vi "Adjust SMU Meas Sense.vi"(7 "Pins":string[](array[string]), 8 "error in (no error)":errorcluster, 10 "Set_Meas_Sense":i32(ring)=1008 items=["Local"=1008, "Remote"=1009], 11 "Semiconductor Module Context":T1) -> (0 "error out":errorcluster, 1 "Measurement:Sense":i32(ring)=1008 items=["Local"=1008, "Remote"=1009], 3 "Semiconductor Module Context Out":T1)   [LabVIEW 2013]
uses:
  <vilib>/NI_TestStand_SemiconductorModule/NI_TestStand_Semiconductor_Module.lvlibp/PinMap/General/SemiconductorModuleContext.ctl
  <vilib>/NI_TestStand_SemiconductorModule/NI_TestStand_Semiconductor_Module.lvlibp/PinMap/DC Power/PinsToNIDCPowerSessions.vi
  <vilib>/NI_TestStand_SemiconductorModule/NI_TestStand_Semiconductor_Module.lvlibp
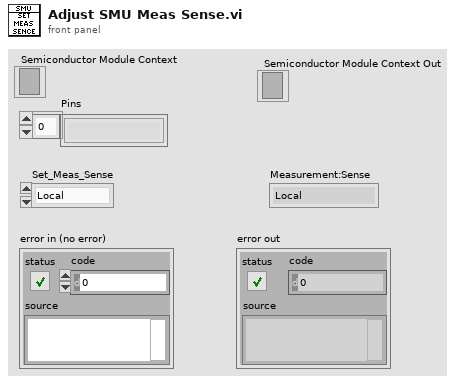
[diagram p1: front panel]
types:
  T1 = typedef "NI_TestStand_Semiconductor_Module.lvlibp/SemiconductorModuleContext.ctl" = refnum<k7>
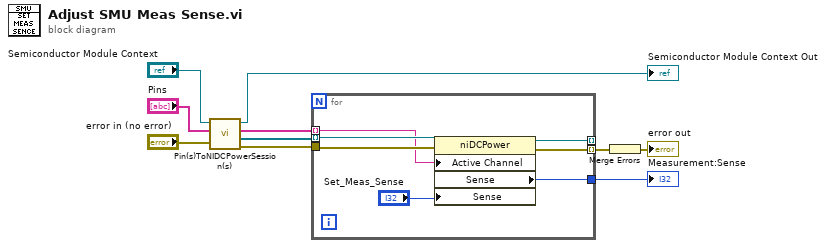
[diagram p0: block diagram]
diagram:
  n1 = call-poly <vilib>:"Pin(s)ToNIDCPowerSession(s).vi"("error in (no error)"="error in (no error)", "Pins"="Pins", "Semiconductor Module Context"="Semiconductor Module Context") -> ("error out"=w10:errorcluster, "Instrument Sessions"=w9:refnum<k15>[], "Channel Lists"=w3:string[], "Semiconductor Module Context Out"=→"Semiconductor Module Context Out":T1)  [unwired: 4 in, 1 out]
  n2 = for {
    tunnel: w10 -> [w17]
    tunnel: w9 -> [w16] mode=indexing
    tunnel: w3 -> [w15] mode=indexing
    tunnel: [w14] -> w5 mode=indexing
    tunnel: [w13] -> _ mode=indexing
    tunnel: [w12] -> w2
    n3 = property class="niDCPower"(reference=w16, error in=w17, "Active Channel"=w15, "Sense"="Set_Meas_Sense") -> (reference out=w13:refnum<k15>, error out=w14:errorcluster, "Sense"=w12:i32)
  }
  "Measurement:Sense" <- w2
  n4 = Merge Errors(w5) -> (→"error out":errorcluster)
